vi "fgv_ngok_global.vi"(7 "cmd":T1, 11 "results":string[](array[string])) -> (3 "results 2":string[](array[string]))   [LabVIEW 2019]
uses:
  _ctrl/rw.ctl
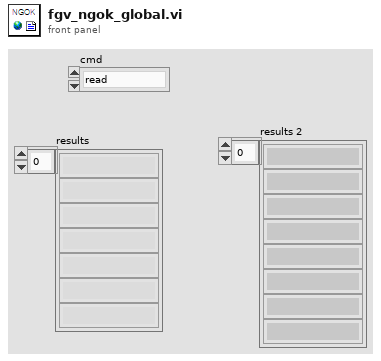
[diagram p1: front panel]
types:
  T1 = typedef "rw.ctl" = enum16{"read", "write"}
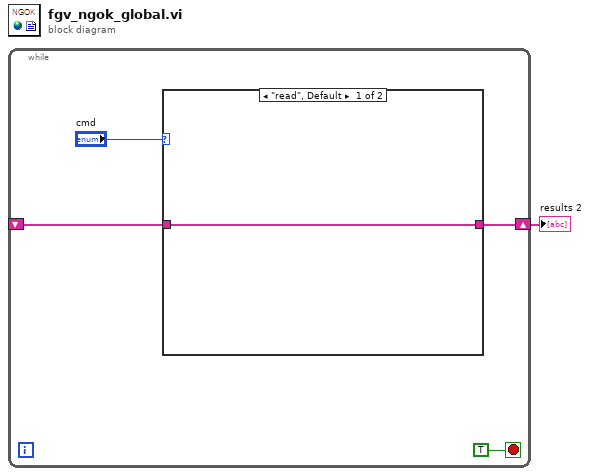
[diagram p0: block diagram]
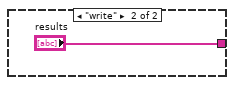
[diagram p2: hidden frame]
diagram:
  n1 = while {
    shift-right: [w3] -> w1
    shift-left: _ -> [w2]
    stop <- TRUE stop-if-true
    n2 = case shown="\"read\", Default" "cmd" {
      tunnel: [w6 "results"] -> w3
      tunnel: w2 -> [w6 _]
      frame "read", Default {
      }
      frame "write" {
      }
    }
  }
  "results 2" <- w1
